vi "RSZVB Select More Ratios.vi"(0 "VISA session":refnum<visa-resource-name>, 1 "Numerator Port Number (1)":i32=1, 2 "Denominator Port Number (1)":i32=1, 5 "Channel (1)":i32=1, 7 "Trace Name (Trc1)":string="Trc1", 9 "Source Port (1: Port 1)":i32=1, 11 "error in (no error)":errorcluster {"code" format="%.0x"}, 12 "Denominator Type (0: a)":i32(ring) items=["a", "b"], 13 "Numerator Type (0: a)":i32(ring) items=["a", "b"]) -> (4 "dup VISA session":refnum<visa-resource-name>, 15 "error out":errorcluster {"code" format="%.0x"})   [LabVIEW 2011]
doc: "This VI select arbitrary ratios of wave quantities, e.g. for different detectors and source ports or more than 2 ports.\n\nAssigns a measurement parameter to an existing trace or creates a trace and assigns a channel number, a name and a measurement parameter to it. The trace is not displayed.\n\nThe notation for ratios and the VIality of the More Ratios dialog is analogous to the definition of S-parameters.\n\nRatio of wave quantities with port numbers and source port numbers (D<no> for drive port; the source port for the numerator and the denominator can be equal or different).\n\nRemote-control command(s):\nCALCulate<Ch>:PARameter:SDEFine '<string>', 'B2D1/A1D1' | 'B1D1/A1D1' | 'B2D1/B1D1' | 'B1D1/B2D1' | ...\nCALCulate<Ch>:PARameter:MEASure '<string>', 'B2D1/A1D1' | 'B1D1/A1D1' | 'B2D1/B1D1' | 'B1D1/B2D1' | ..."
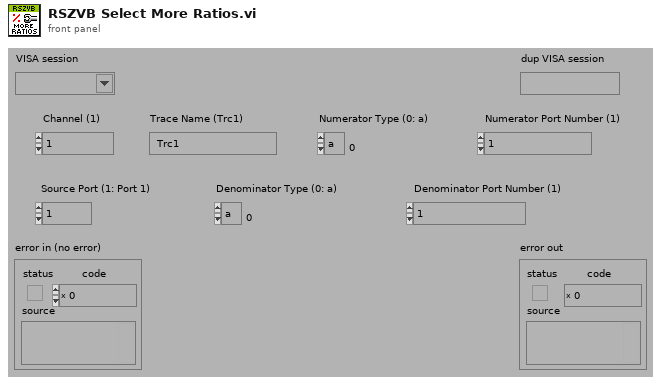
[diagram p1: front panel]
types:
  T1 = cluster{"Error Checking (T: On)":bool, "Installed Options":string[], "Data Valid?":bool, "Ports":i32, "Model":string[], "Option Checking (T: On)":bool}
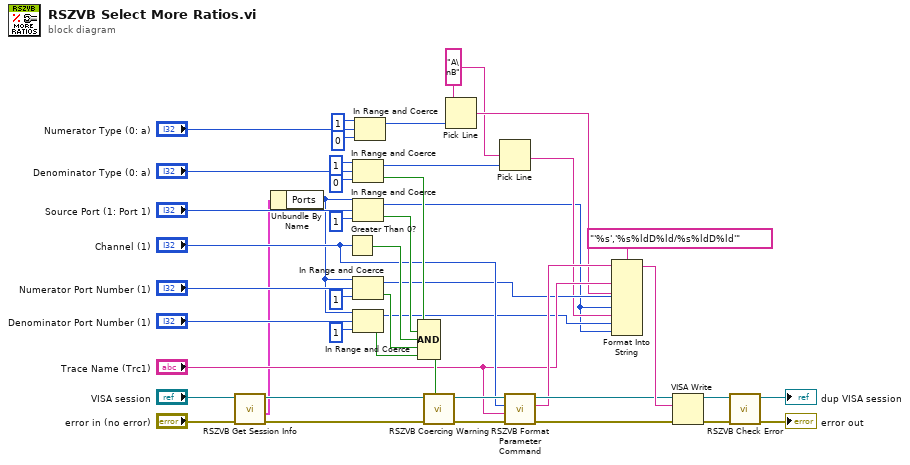
[diagram p0: block diagram]
diagram:
  w10 = "A\nB"
  n1 = call "RSZVB Get Session Info.vi"("error in (no error)"="error in (no error)", "VISA session"="VISA session") -> ("error out"=w4:errorcluster, "Session Info"=w2:T1, "dup VISA session"=w3:refnum<visa-resource-name>)  [unwired: 7 in]
  n2 = Unbundle By Name(w2) -> ("Ports"=w1:i32)
  n3 = Greater Than 0?(x="Channel (1)") -> (x > 0?=w27:bool)
  n4 = In Range and Coerce(upper limit=1, x="Denominator Type (0: a)", lower limit=0) -> (coerced(x)=w30:i32, In Range?=w29:bool)
  n5 = In Range and Coerce(upper limit=w1, x="Source Port (1: Port 1)", lower limit=1) -> (coerced(x)=w7:i32, In Range?=w28:bool)
  n6 = In Range and Coerce(upper limit=w1, x="Numerator Port Number (1)", lower limit=1) -> (coerced(x)=w12:i32, In Range?=w26:bool)
  n7 = In Range and Coerce(upper limit=w1, x="Denominator Port Number (1)", lower limit=1) -> (coerced(x)=w9:i32, In Range?=w25:bool)
  n8 = In Range and Coerce(upper limit=1, x="Numerator Type (0: a)", lower limit=0) -> (coerced(x)=w13:i32)  [unwired: 1 out]
  n9 = Compound Arithmetic op=AND(w29, w28, w27, w26, w25) -> (w41:bool)
  n10 = call "RSZVB Coercing Warning.vi"("In Range?"=w41, "error in (no error)"=w4, "VISA session"=w3) -> ("error out"=w38:errorcluster, "dup VISA session"=w37:refnum<visa-resource-name>)  [unwired: 7 in]
  n11 = Pick Line(multi-line string=w10, line index=w13) -> (output string=w11:string)  [unwired: 1 in]
  n12 = Pick Line(multi-line string=w10, line index=w30) -> (output string=w8:string)  [unwired: 1 in]
  n13 = call "RSZVB Format Parameter Command.vi"("error in (no error)"=w38, "Trace Name (Trc1)"="Trace Name (Trc1)", "Channel (1)"="Channel (1)", "VISA session"=w37) -> ("error out"=w39:errorcluster, "Buffer"=w34:string, "dup VISA session"=w36:refnum<visa-resource-name>)  [unwired: 5 in]
  n14 = Format Into String(format string="'%s','%s%ldD%ld/%s%ldD%ld'", initial string=w34, "Trace Name (Trc1)", w11, w12, w7, w8, w9, w7) -> (resulting string=w40:string)  [unwired: 1 in, 1 out]
  n15 = VISA Write(VISA resource name=w36, write buffer=w40, error in (no error)=w39) -> (VISA resource name out=w42:refnum<visa-resource-name>, error out=w43:errorcluster)  [unwired: 1 out]
  n16 = call "RSZVB Check Error.vi"("error in (no error)"=w43, "VISA session"=w42) -> ("error out"=→"error out":errorcluster, "dup VISA session"=→"dup VISA session":refnum<visa-resource-name>)  [unwired: 8 in]
